vi "exnSpectralBlock clear array magnitudes.vi"(1 "magnitudes in":cluster{"f0":dbl, "df":dbl, "magnitude":dbl[]}[](array[cluster]) {"magnitude" format="%.2p"; "f0" format="%.2p"; "df" format="%.2p"}) -> (0 "magnitudes out":cluster{"f0":dbl, "df":dbl, "magnitude":dbl[]}[](array[cluster]) {"magnitude" format="%.2p"; "f0" format="%.2p"; "df" format="%.2p"})   [LabVIEW 2017]
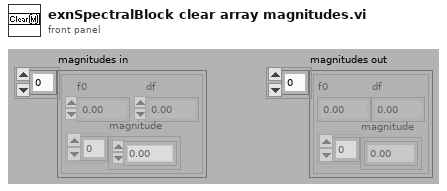
[diagram p1: front panel]
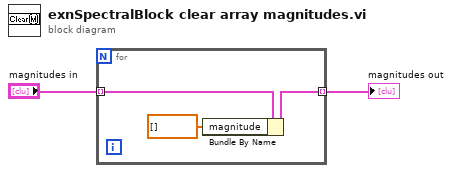
[diagram p0: block diagram]
diagram:
  n1 = for {
    tunnel: "magnitudes in" -> [w4] mode=indexing
    tunnel: [w3] -> w1 mode=indexing
    n2 = Bundle By Name(cluster=w4, "magnitude"=dbl[] []) -> (w3:cluster{"f0":dbl, "df":dbl, "magnitude":dbl[]})
  }
  "magnitudes out" <- w1
